vi "tab control exp 3.vi"() -> ()   [LabVIEW 2024]
panel:
  in  "Tab Control":T1(tab)
  in  "Numeric 2":dbl
  in  "Numeric 1":dbl
  out "Waveform  Graph":dynamicdata(graph)
  in  "Frequency":dbl(knob) scale=0.0..1000.0
  in  "Amplitude":dbl(knob) scale=0.0..10.0
  in  "Array 5":dbl[](array[numeric])
  in  "Array 4":dbl[](array[numeric])
  out "Output Waveform":dynamicdata(graph)
  in  "Cluster 2":T2
  in  "Cluster":T2
  out "Waveform Chart":dynamicdata(graph)
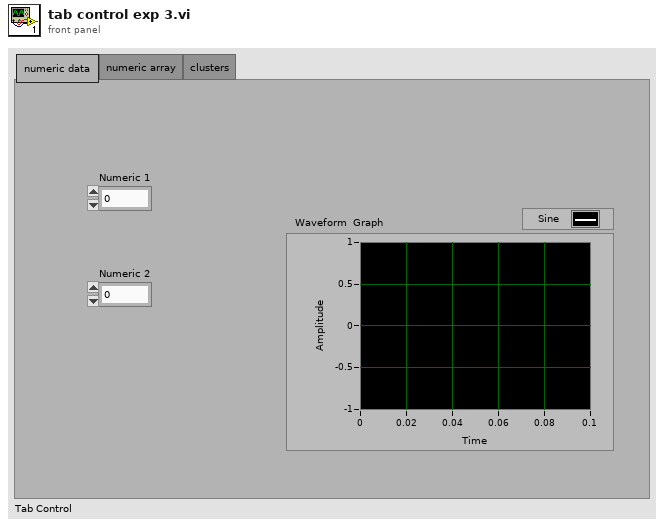
[diagram p1: front panel]
types:
  T1 = enum32{"numeric data ", "numeric array", "clusters"}
  T2 = cluster{"Numeric":dbl, "Boolean":bool, "String":string}
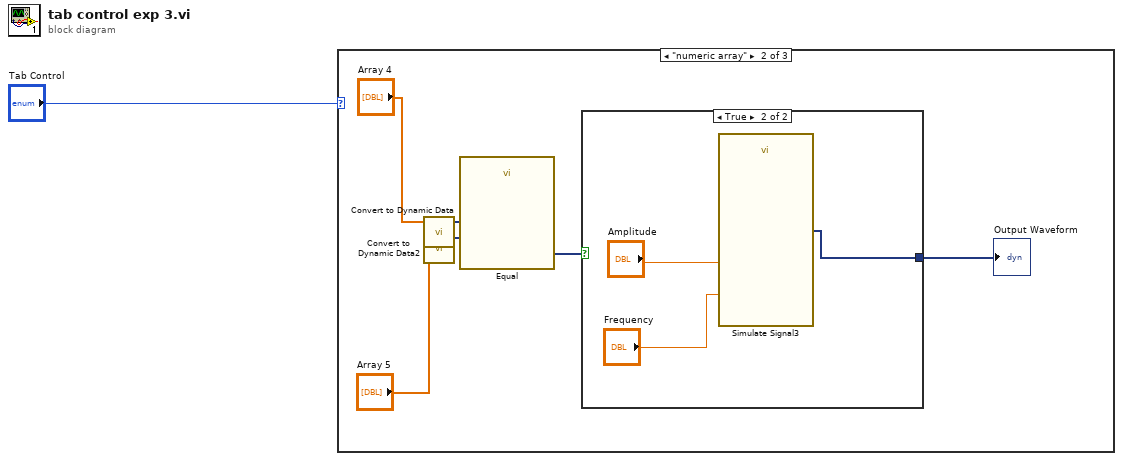
[diagram p0: block diagram]
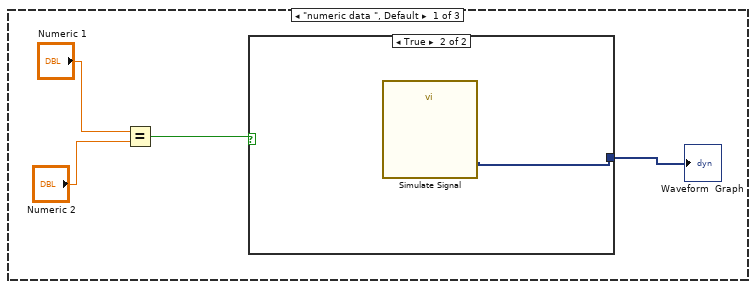
[diagram p2: hidden frame]
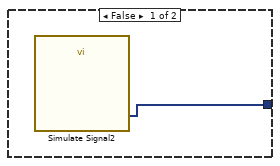
[diagram p3: hidden frame]
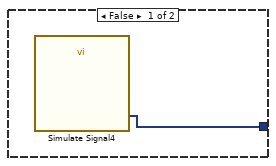
[diagram p4: hidden frame]
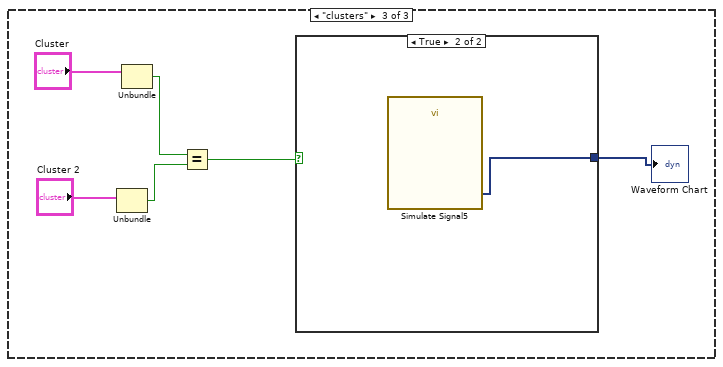
[diagram p5: hidden frame]
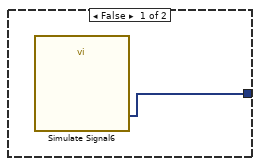
[diagram p6: hidden frame]
diagram:
  n1 = case shown="\"numeric array\"" "Tab Control" {
    frame "numeric data ", Default {
      n2 = Equal?(x="Numeric 1", y="Numeric 2") -> (x = y?=w2:bool)
      n3 = case shown="True" w2 {
        tunnel: [w6 w7] -> w5
        frame False {
          n4 = call "Simulate Signal2"() -> ("DC"=w6:dynamicdata)  [unwired: 14 in, 1 out]
        }
        frame True {
          n5 = call "Simulate Signal"() -> ("Sine"=w7:dynamicdata)  [unwired: 14 in, 1 out]
        }
      }
      "Waveform  Graph" <- w5
    }
    frame "numeric array" {
      n6 = call "Convert to Dynamic Data"("Array"="Array 4") -> ("Dynamic Data Type"=w10:dynamicdata)  [unwired: 3 in]
      n7 = call "Convert to Dynamic Data2"("Array"="Array 5") -> ("Dynamic Data Type"=w8:dynamicdata)  [unwired: 3 in]
      n8 = call "Equal"("Operand 2"=w8, "Operand 1"=w10) -> ("Result"=w12:dynamicdata)  [unwired: 8 in, 1 out]
      n9 = case shown="True" w12 {
        tunnel: [w14 w15] -> w13
        frame False {
          n10 = call "Simulate Signal4"() -> ("DC"=w14:dynamicdata)  [unwired: 14 in, 1 out]
        }
        frame True {
          n11 = call "Simulate Signal3"("Frequency"="Frequency", "Amplitude"="Amplitude") -> ("Sine"=w15:dynamicdata)  [unwired: 12 in, 1 out]
        }
      }
      "Output Waveform" <- w13
    }
    frame "clusters" {
      n12 = Unbundle("Cluster 2") -> ("Boolean"=w20:bool)  [unwired: 2 out]
      n13 = Unbundle("Cluster") -> ("Boolean"=w19:bool)  [unwired: 2 out]
      n14 = Equal?(x=w19, y=w20) -> (x = y?=w23:bool)
      n15 = case shown="True" w23 {
        tunnel: [w24 w25] -> w18
        frame False {
          n16 = call "Simulate Signal6"() -> ("DC"=w24:dynamicdata)  [unwired: 14 in, 1 out]
        }
        frame True {
          n17 = call "Simulate Signal5"() -> ("Sine"=w25:dynamicdata)  [unwired: 14 in, 1 out]
        }
      }
      "Waveform Chart" <- w18
    }
  }
